vi "MeanArraySpacing.vi"(6 "Technique":enum16{"Max-Min", "Mean delta"}(ring), 11 "Array":dbl[](array[numeric])) -> (3 "Mean Spacing":dbl)   [LabVIEW 2013]
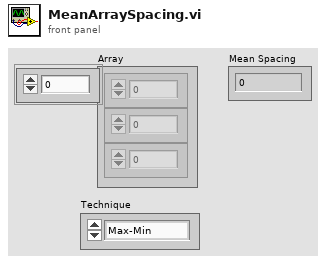
[diagram p1: front panel]
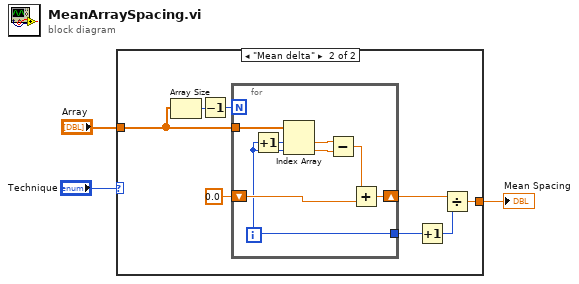
[diagram p0: block diagram]
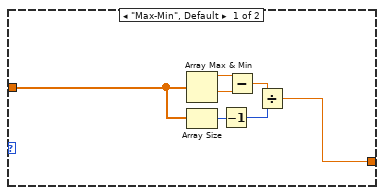
[diagram p2: hidden frame]
diagram:
  n1 = case shown="\"Mean delta\"" "Technique" {
    tunnel: [w10 w17] -> w3
    tunnel: "Array" -> [w5 w16]
    frame "Max-Min", Default {
      n2 = Array Max & Min(array=w5) -> (max value=w6:dbl, min value=w7:dbl)  [unwired: 2 out]
      n3 = Array Size(array=w5) -> (size(s)=w9:i32)
      n4 = Decrement(x=w9) -> (x-1=w4:i32)
      n5 = Subtract(x=w6, y=w7) -> (x-y=w8:dbl)
      n6 = Divide(x=w8, y=w4) -> (x/y=w10:dbl)
    }
    frame "Mean delta" {
      n7 = Array Size(array=w16) -> (size(s)=w15:i32)
      n8 = Decrement(x=w15) -> (x-1=w14:i32)
      n9 = for {
        N: w14 -> [_]
        shift-right: [w23] -> w18
        shift-left: 0.0 -> [w24]
        tunnel: [w19] -> w13
        tunnel: w16 -> [w22]
        i -> [w19]
        n10 = Increment(x=w19) -> (x+1=w20:i32)
        n11 = Index Array(array=w22, index #1=w20, index #2=w19) -> (element #1=w26:dbl, element #2=w25:dbl)
        n12 = Subtract(x=w26, y=w25) -> (x-y=w21:dbl)
        n13 = Add(x=w21, y=w24) -> (x+y=w23:dbl)
      }
      n14 = Increment(x=w13) -> (x+1=w12:i32)
      n15 = Divide(x=w18, y=w12) -> (x/y=w17:dbl)
    }
  }
  "Mean Spacing" <- w3
